vi "VI Tester Project API Open and Run All Tests.vi"(8 "error in":errorcluster, 11 "Object":T1) -> (0 "error out":errorcluster)   [LabVIEW 2009]
uses:
  VITester Project Item Ref.ctl
  VI Tester Project API Method Selector - Enum.ctl
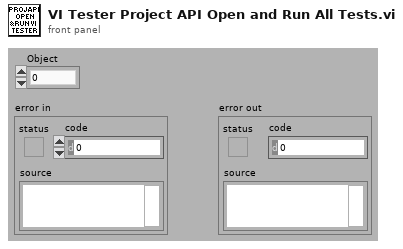
[diagram p1: front panel]
types:
  T1 = typedef "VITester Project Item Ref.ctl" = u64
  T2 = typedef "VI Tester Project API Method Selector - Enum.ctl" = enum16{"Open VI Tester", "Run All Tests", "Create New TestCase", "Create New TestSuite"}
  T3 = enum32{"Bad", "Idle", "Run top level", "Running"}
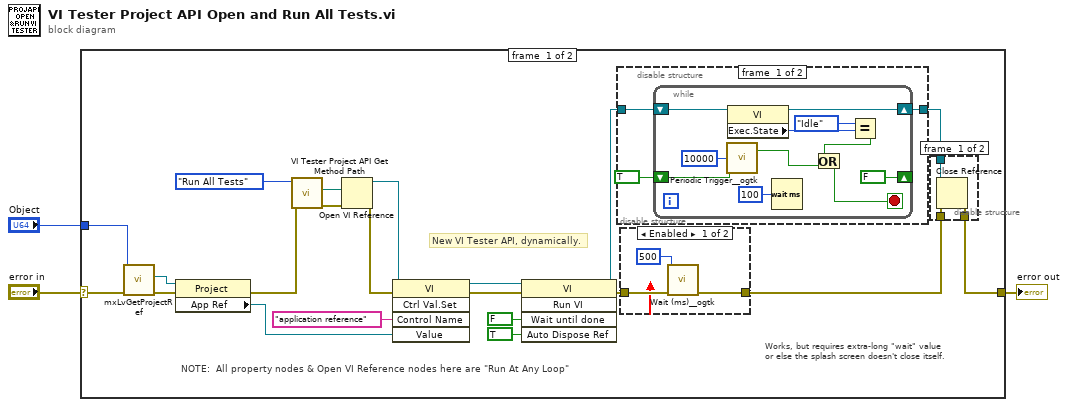
[diagram p0: block diagram]
diagram:
  n1 = case shown="No Error" "error in" {
    selector: "error in" -> [w9 w48]
    tunnel: [w24 w48] -> w3
    tunnel: "Object" -> [w21 _]
    frame #0 {
      # "Works, but requires extra-long \"wait\" value\nor else the splash screen doesn't close itself."
      # "NOTE:  All property nodes & Open VI Reference nodes here are \"Run At Any Loop\""
      # "New VI Tester API, dynamically."
      n2 = call "mxLvGetProjectRef.vi"("error in"=w9, "Item"=w21) -> ("error out"=w11:errorcluster, "Project Refnum"=w12:refnum<vi>)  [unwired: 7 in, 1 out]
      n3 = property class="Project"(reference=w12, error in=w11) -> (error out=w7:errorcluster, "App Ref"=w10:refnum<vi>)  [unwired: 1 out]
      n4 = call "VI Tester Project API Get Method Path.vi"("error in (no error)"=w7, "Project API Method"=VI_Tester_Project_API_Method_Selector_-_Enum."Run All Tests") -> ("error out"=w6:errorcluster, "Path to VI Tester Project API Proxy VI"=w22:path)  [unwired: 8 in]
      n5 = Open VI Reference(vi path=w22, error in (no error)=w6) -> (vi reference=w15:refnum<vi>, error out=w17:errorcluster)  [unwired: 4 in]
      n6 = invoke class="VI" method="Ctrl Val.Set"(reference=w15, error in=w17, "Control Name"="application reference", "Value"=w10) -> (reference out=w14:refnum<vi>, error out=w16:errorcluster)  [unwired: 1 in, 3 out]
      n7 = invoke class="VI" method="Run VI"(reference=w14, error in=w16, "Wait until done"=FALSE ("Wait Until Done"), "Auto Dispose Ref"=TRUE ("Auto Dispose Reference")) -> (reference out=w4:refnum<vi>, error out=w18:errorcluster)  [unwired: 1 in, 3 out]
      n8 = disable-structure shown="Enabled" {
        disable-tunnel: [w30 w43] -> w5
        disable-tunnel: w4 -> [w29 w43]
        frame #0 {
          n9 = while {
            shift-right: [FALSE] -> _
            shift-left: TRUE -> [w40]
            shift-right: [w33] -> w30
            shift-left: w29 -> [w42]
            stop <- w34 stop-if-true
            n10 = call <userlib>:"Periodic Trigger__ogtk.vi"("time (ms)"=u32 10000, "reset"=w40) -> ("Triggered"=w35:bool)  [unwired: 11 in, 2 out]
            n11 = property class="VI"(reference=w42) -> (reference out=w33:refnum<vi>, "Exec.State"=w38:T3)  [unwired: 1 in, 1 out]
            n12 = Wait (ms)(milliseconds to wait=u32 100) -> ()  [unwired: 1 out]
            n13 = Equal?(x=T3."Idle", y=w38) -> (x = y?=w36:bool)
            n14 = Or(x=w36, y=w35) -> (x .or. y?=w34:bool)
          }
        }
        frame #1 {
        }
      }
      n15 = disable-structure shown="Enabled" {
        disable-tunnel: [w46 w47] -> w23
        disable-tunnel: w18 -> [w45 w47]
        frame #0 {
          n16 = call <userlib>:"Wait (ms)__ogtk.vi"("error in (no error)"=w45, "milliseconds to wait"=u32 500) -> ("error out"=w46:errorcluster)  [unwired: 8 in, 1 out]
        }
        frame #1 {
        }
      }
      n17 = disable-structure shown="Enabled" {
        disable-tunnel: [w27 w28] -> w24
        disable-tunnel: w23 -> [w26 w28]
        disable-tunnel: w5 -> [w25 _]
        frame #0 {
          n18 = Close Reference(reference=w25, error in (no error)=w26) -> (error out=w27:errorcluster)
        }
        frame #1 {
        }
      }
    }
    frame #1 {
    }
  }
  "error out" <- w3
